vi "Init Device.vi"(7 "Layout Ref":refnum<vi>, 8 "error in (no error)":errorcluster, 10 "Chan# Array":i32[](array[numeric]), 11 "PTS-via-PB in":refnum<class "PTS-via-PB.lvclass">) -> (0 "error out":errorcluster, 3 "PTS-via-PB out":refnum<class "PTS-via-PB.lvclass">)   [LabVIEW 2013, in "PTS-via-PB.lvclass"]
doc: "Initialize the correct columns and their default appearance.\nUse the front panel to change default appearance of the device in the Add/Manage devices.\n\nOpen a specific device implementation for details."
uses:
  PTS-via-PB.lvclass
  TypeDefs/ColumnAppearCluster.ctl
  ColumnVIs/Column/Column.lvclass
panel:
  in  "Freq Col Defaults":T1={"Column Name"="RF Freq.", "Width"=30, "Bkgd"=[16448250], "Text"=[0]}
  in  "SpinAPI Path":path=path "C:/SpinCore/SpinAPI/dll/spinapi.dll"
  in  "Board Number":i32=1 max=256 step=1
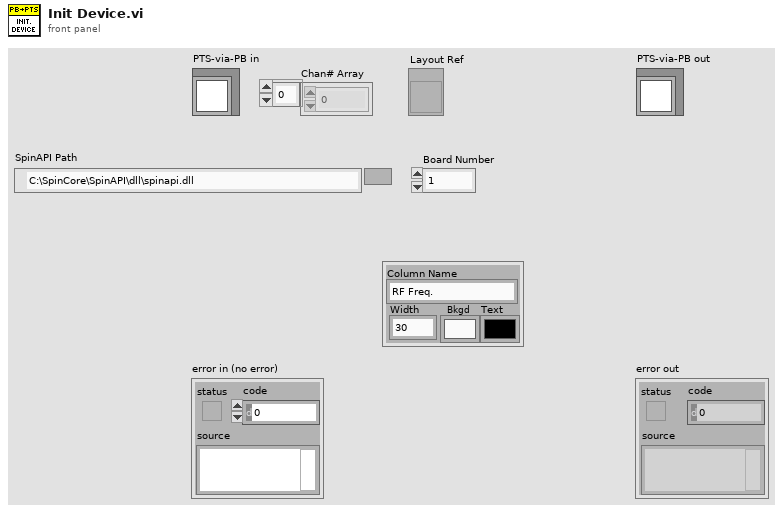
[diagram p1: front panel]
types:
  T1 = typedef "ColumnAppearCluster.ctl" = cluster{"Column Name":string, "Width":u32, "Bkgd":u32[], "Text":u32[]}
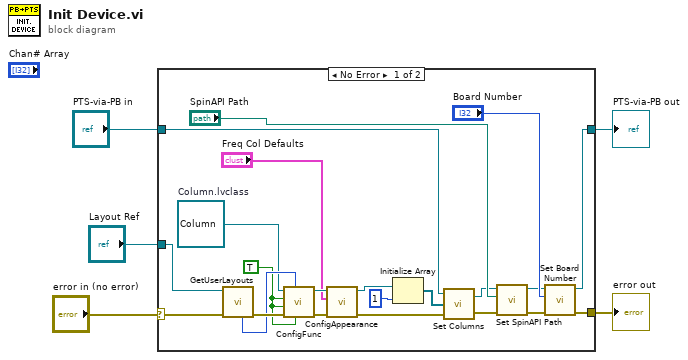
[diagram p0: block diagram]
diagram:
  n1 = case shown="No Error" "error in (no error)" {
    selector: "error in (no error)" -> [w20 w28]
    tunnel: "PTS-via-PB in" -> [w8 w29]
    tunnel: [w13 w29] -> w1
    tunnel: [w14 w28] -> w2
    tunnel: "Layout Ref" -> [w23 _]
    frame No Error {
      w19 = refnum<class "Column.lvclass"> refnum  # Column.lvclass
      w6 = TRUE ("Disableable? (True)")
      n2 = call "GetUserLayouts.vi"("error in (no error)"=w20, "Layout Ring Refnum"=w23) -> ("error out"=w22:errorcluster, "Num User Layouts"=w21:i32)  [unwired: 5 in, 3 out]
      n3 = call "ConfigFunc.vi"("isRampable? (True"=w6, "Num Layouts (ignored)"=w21, "error in (no error)"=w22, "isVariable? (True)"=w6, "Disableable? (True)"=w6, "Column in"=w19) -> ("error out"=w26:errorcluster, "Column out"=w25:refnum<class "Column.lvclass">)  [unwired: 4 in]
      n4 = call "ConfigAppearance.vi"("error in (no error)"=w26, "Column Appearance"="Freq Col Defaults", "Column in"=w25) -> ("error out"=w10:errorcluster, "Column out"=w24:refnum<class "Column.lvclass">)  [unwired: 7 in]
      n5 = Initialize Array(w24, 1 ("dimension size")) -> (w7:refnum<class "Column.lvclass">[])
      n6 = call-dynamic "Set Columns.vi"("error in (no error)"=w10, "Columns in"=w7, "Pulseblaster in"=w8) -> ("error out"=w11:errorcluster, "Pulseblaster out"=w9:refnum<class "PTS-via-PB.lvclass">)  [unwired: 1 in]
      n7 = call-dynamic "Set SpinAPI Path.vi"("error in (no error)"=w11, "SpinAPI Path"="SpinAPI Path", "Pulseblaster in"=w9) -> ("error out"=w15:errorcluster, "Pulseblaster out"=w16:refnum<class "PTS-via-PB.lvclass">)  [unwired: 7 in]
      n8 = call-dynamic "Set Board Number.vi"("error in (no error)"=w15, "Board Number"="Board Number", "Pulseblaster in"=w16) -> ("error out"=w14:errorcluster, "Pulseblaster out"=w13:refnum<class "PTS-via-PB.lvclass">)  [unwired: 7 in]
    }
    frame Error {
    }
  }
  "error out" <- w2
  "PTS-via-PB out" <- w1
